vi "SetPivot.vi"(8 "error in (no error)":errorcluster, 11 "Settings.PivotPoint":T1) -> (0 "error out":errorcluster)   [LabVIEW 2020]
panel:
  out "Controller error":bool
  in  "Pivot point coordinates":cluster{"R":dbl, "S":dbl, "T":dbl} {"T" format="%.4f"; "S" format="%.4f"; "R" format="%.4f"}
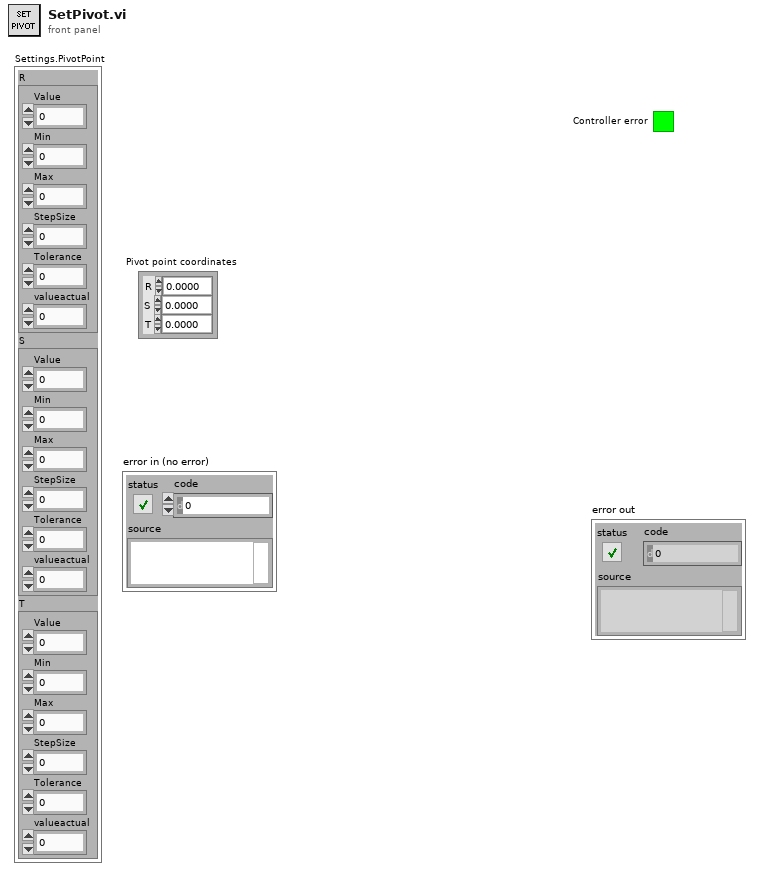
[diagram p1: front panel]
types:
  T1 = cluster{"R":cluster{"Value":dbl, "Min":dbl, "Max":dbl, "StepSize":dbl, "Tolerance":dbl, "valueactual":dbl}, "S":cluster{"Value":dbl, "Min":dbl, "Max":dbl, "StepSize":dbl, "Tolerance":dbl, "valueactual":dbl}, "T":cluster{"Value":dbl, "Min":dbl, "Max":dbl, "StepSize":dbl, "Tolerance":dbl, "valueactual":dbl}}
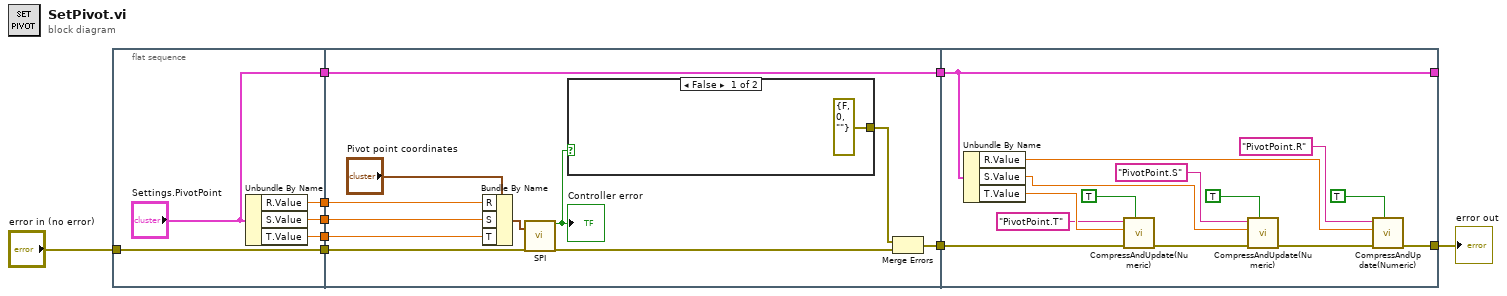
[diagram p0: block diagram]
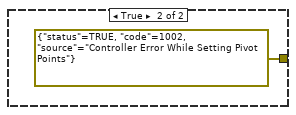
[diagram p2: hidden frame]
diagram:
  n1 = flat-sequence {
    tunnel: [w14] -> w9
    tunnel: [w13] -> w8
    tunnel: [w12] -> w7
    tunnel: ["Settings.PivotPoint"] -> w6
    tunnel: [w10] -> w5
    tunnel: "error in (no error)" -> [w10]
    tunnel: w9 -> [w23]
    tunnel: w8 -> [w22]
    tunnel: w7 -> [w21]
    tunnel: w6 -> [w17]
    tunnel: w5 -> [w16]
    tunnel: [w18] -> w3
    tunnel: [w17] -> w2
    tunnel: [w41] -> _
    tunnel: w3 -> [w39]
    tunnel: w2 -> [w41]
    tunnel: [w28] -> w1
    frame #0 {
      n2 = Unbundle By Name("Settings.PivotPoint") -> ("R.Value"=w14:dbl, "S.Value"=w13:dbl, "T.Value"=w12:dbl)
    }
    frame #1 {
      n3 = Bundle By Name(cluster="Pivot point coordinates", "R"=w23, "S"=w22, "T"=w21) -> (w24:cluster{"R":dbl, "S":dbl, "T":dbl})
      n4 = call "SPI.vi"("Pivot point coordinates"=w24, "error in"=w16) -> ("Controller error"=w20:bool, "error out"=w15:errorcluster)  [unwired: 16 in]
      "Controller error" <- w20
      n5 = case shown="False" w20 {
        tunnel: [errorcluster {"status"=FALSE, "code"=0, "source"=""} ("error out") errorcluster {"status"=TRUE, "code"=1002, "source"="Controller Error While Setting Pivot Points"} ("error out")] -> w19
        frame False {
        }
        frame True {
        }
      }
      n6 = Merge Errors(w19, w15) -> (w18:errorcluster)
    }
    frame #2 {
      n7 = Unbundle By Name(w41) -> ("R.Value"=w31:dbl, "S.Value"=w32:dbl, "T.Value"=w38:dbl)
      n8 = call "CompressAndUpdate(Numeric).vi"("force CVT update (false)"=TRUE, "error in"=w39, "Numeric"=w38, "command or variable name"="PivotPoint.T") -> ("error out"=w30:errorcluster)  [unwired: 7 in]
      n9 = call "CompressAndUpdate(Numeric).vi"("force CVT update (false)"=TRUE, "error in"=w30, "Numeric"=w32, "command or variable name"="PivotPoint.S") -> ("error out"=w29:errorcluster)  [unwired: 7 in]
      n10 = call "CompressAndUpdate(Numeric).vi"("force CVT update (false)"=TRUE, "error in"=w29, "Numeric"=w31, "command or variable name"="PivotPoint.R") -> ("error out"=w28:errorcluster)  [unwired: 7 in]
    }
  }
  "error out" <- w1
